vi "Counter_LRH.vi"() -> ()   [LabVIEW 2013]
uses:
  <vilib>/eio/EIONode/EIONode.xnode
  <instrlib>/_niInstr/Basic Elements/v1/FPGA/niInstr Basic Elements v1 FPGA.lvlib
  <instrlib>/_niInstr/Basic Elements/v1/FPGA/Private/Count Up U64.vi
  <vilib>/rvi/eio/common/nirviEmuTemplateMethod_errors.vi
panel:
  out "count out 9":u64
  out "count out 8":u64
  out "count out 7":u64
  out "count out 6":u64
  out "count out 5":u64
  out "count out 4":u64
  out "count out 3":u64
  in  "Trigger":bool
  out "Zeit läuft":bool
  in  "Ablaufzeit":i64=10
  out "Boolean":bool
  in  "reset":bool
  out "count out 2":u64
  out "count out 1":u64
  in  "stop":bool
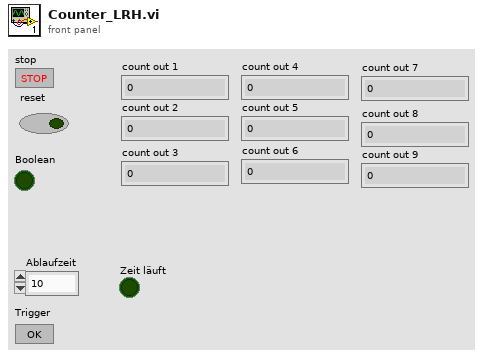
[diagram p1: front panel]
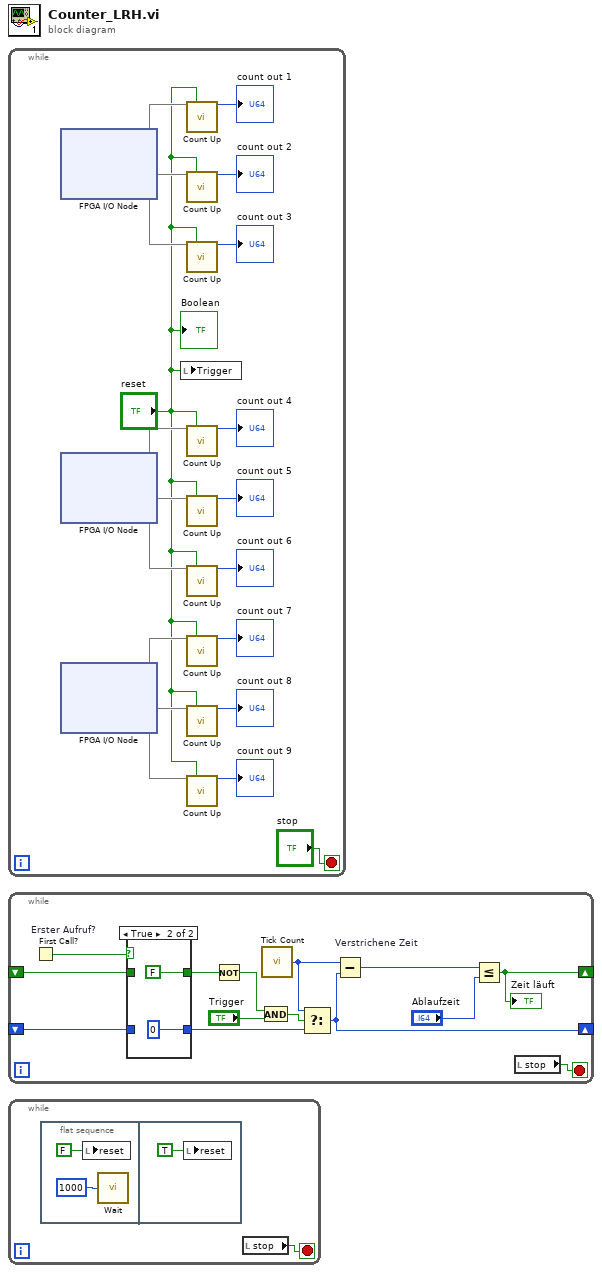
[diagram p0: block diagram]
diagram:
  n1 = while {
    stop <- "stop" stop-if-true
    n2 = xnode "FPGA I/O Node"() -> ("Mod1/DI0"=w20, "Mod1/DI1"=w19, "Mod1/DI2"=w15)  [unwired: 3 in, 3 out]
    n3 = xnode "FPGA I/O Node"() -> ("Mod2/DI0"=w13, "Mod2/DI1"=w12, "Mod2/DI2"=w11)  [unwired: 3 in, 3 out]
    n4 = xnode "FPGA I/O Node"() -> ("Mod3/DI0"=w7, "Mod3/DI1"=w6, "Mod3/DI2"=w5)  [unwired: 3 in, 3 out]
    n5 = local write "Trigger"("reset") -> ()
    n6 = call-poly <instrlib>:"Count Up.vi"("increment"=w20, "reset"="reset") -> ("count out"=→"count out 1":u64)  [unwired: 13 in]
    n7 = call-poly <instrlib>:"Count Up.vi"("increment"=w19, "reset"="reset") -> ("count out"=→"count out 2":u64)  [unwired: 13 in]
    n8 = call-poly <instrlib>:"Count Up.vi"("increment"=w15, "reset"="reset") -> ("count out"=→"count out 3":u64)  [unwired: 13 in]
    n9 = call-poly <instrlib>:"Count Up.vi"("increment"=w13, "reset"="reset") -> ("count out"=→"count out 4":u64)  [unwired: 13 in]
    n10 = call-poly <instrlib>:"Count Up.vi"("increment"=w12, "reset"="reset") -> ("count out"=→"count out 5":u64)  [unwired: 13 in]
    n11 = call-poly <instrlib>:"Count Up.vi"("increment"=w11, "reset"="reset") -> ("count out"=→"count out 6":u64)  [unwired: 13 in]
    n12 = call-poly <instrlib>:"Count Up.vi"("increment"=w7, "reset"="reset") -> ("count out"=→"count out 7":u64)  [unwired: 13 in]
    n13 = call-poly <instrlib>:"Count Up.vi"("increment"=w6, "reset"="reset") -> ("count out"=→"count out 8":u64)  [unwired: 13 in]
    n14 = call-poly <instrlib>:"Count Up.vi"("increment"=w5, "reset"="reset") -> ("count out"=→"count out 9":u64)  [unwired: 13 in]
    "Boolean" <- "reset"
  }
  n15 = while {
    shift-right: [w25] -> _
    shift-left: _ -> [w29]
    shift-right: [w32] -> _
    shift-left: _ -> [w30]
    stop <- w21 stop-if-true
    n16 = First Call? "Erster Aufruf?"() -> (First Call?: T/F=w31:bool)
    n17 = case shown="True" w31 {
      tunnel: w30 -> [w36 _]
      tunnel: w29 -> [w35 _]
      tunnel: [w36 FALSE] -> w26
      tunnel: [w35 i64 0] -> w28
      frame False {
      }
      frame True {
      }
    }
    n18 = Not(x=w26) -> (.not. x?=w27:bool)
    n19 = And(x=w27, y="Trigger") -> (x .and. y?=w33:bool)
    n20 = call "Tick Count"() -> ("Tick Count(mSec)"=w22:u32)
    n21 = Select(t=w22, s=w33, f=w28) -> (s? t:f=w25:i64)
    n22 = Subtract "Verstrichene Zeit"(x=w22, y=w25) -> (x-y=w24:i64)
    n23 = Less Or Equal?(x=w24, y="Ablaufzeit") -> (x <= y?=w32:bool)
    "Zeit läuft" <- w32
    n24 = local read "stop"() -> (w21:bool)
  }
  n25 = while {
    stop <- w39 stop-if-true
    n26 = flat-sequence {
      frame #0 {
        n27 = local write "reset"(FALSE) -> ()
        n28 = call "Wait"("Count(mSec)"=u32 1000) -> ()  [unwired: 1 out]
      }
      frame #1 {
        n29 = local write "reset"(TRUE) -> ()
      }
    }
    n30 = local read "stop"() -> (w39:bool)
  }
